vi "3_ReadDatatoWaveform.vi"(8 "error in (no error)":errorcluster, 11 "file path (IN)":path) -> (0 "error out":errorcluster, 2 "Waveform Graph":waveform(dbl)[](graph), 3 "file path (OUT)":path, 4 "dt":dbl, 5 "Ch 2 Data":dbl[](array[numeric]), 6 "Ch 3 Data":dbl[](array[numeric]), 7 "Ch 1 Data":dbl[](array[numeric]))   [LabVIEW 2020]
uses:
  <vilib>/Utility/file.llb/Read Delimited Spreadsheet (string).vi
  <vilib>/Utility/file.llb/Read Delimited Spreadsheet (DBL).vi
panel:
  out "Spread Sheet Display":string[][](array[string])
  out "Data Display":dbl[][](array[numeric])
  # "Channel 1"
  # "Channel 2"
  # "Channel 3"
  # "C:\\Users\\zbmbdt\\Desktop\\Assignment\\Project1_AC Module\\LabVIEW_Project_AC_Module\\1_ALL_VI\\GRAPH_11_30\\graphdata.csv"
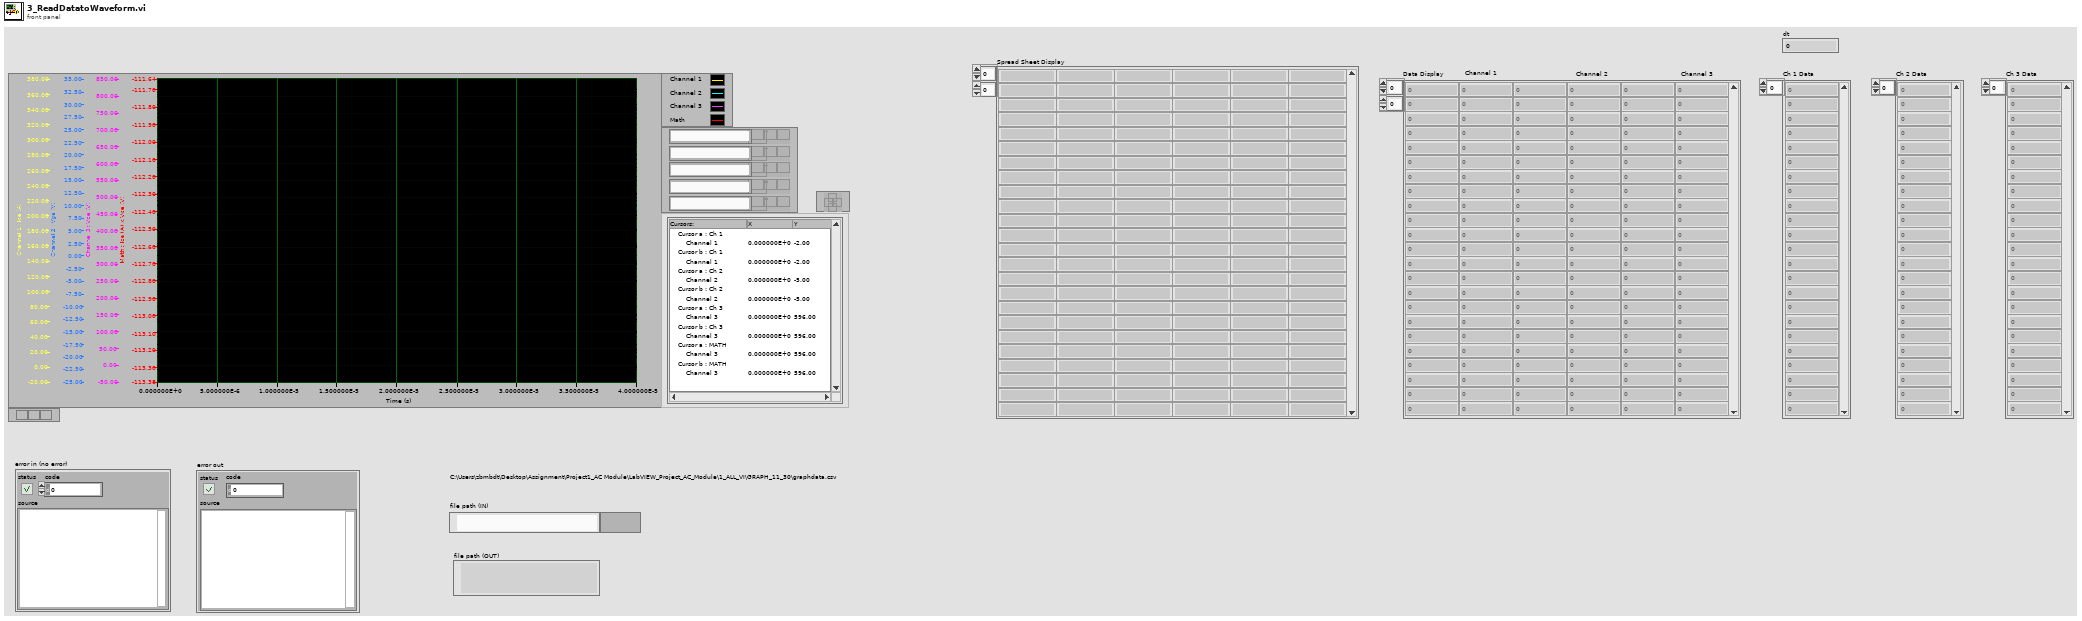
[diagram p1: front panel]
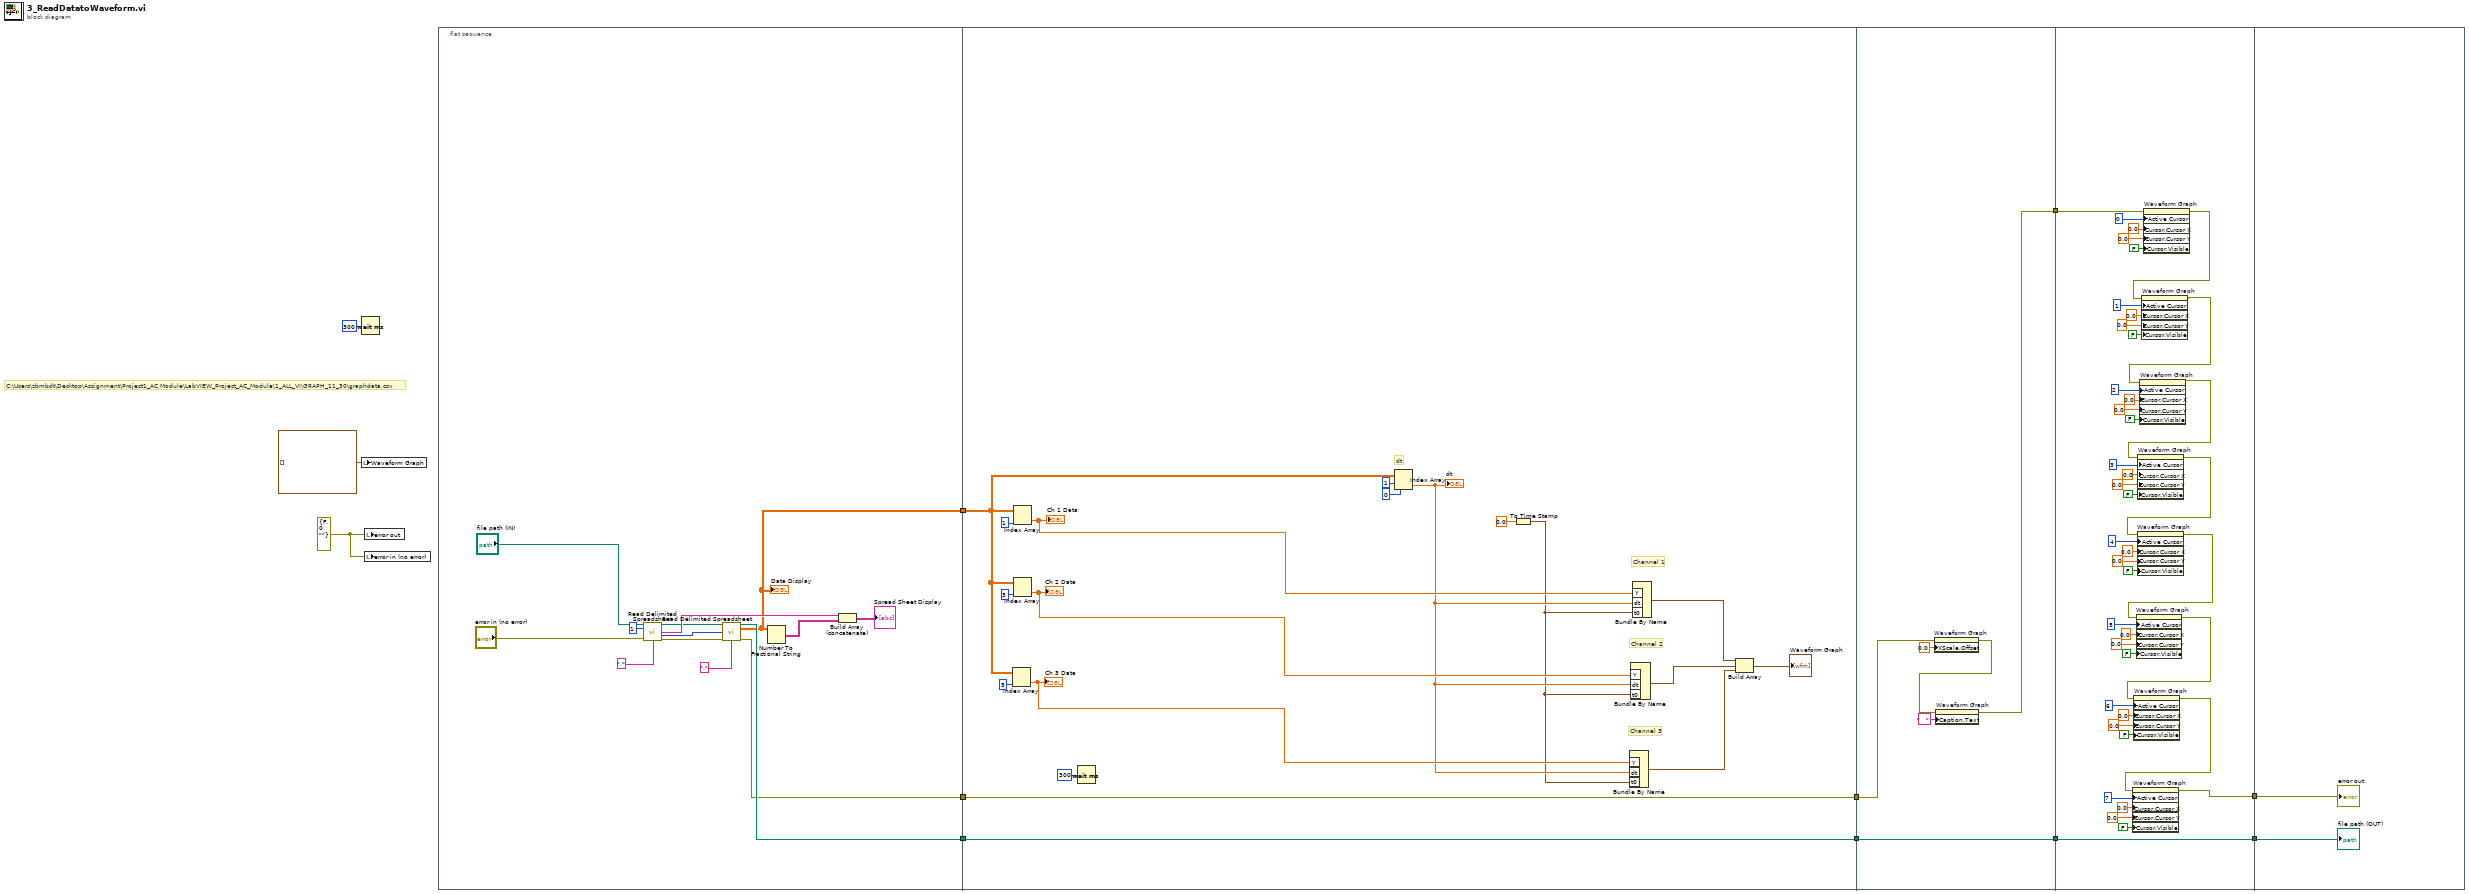
[diagram p0: block diagram]
diagram:
  w2 = errorcluster {"status"=FALSE, "code"=0, "source"=""} ("error out")
  # "C:\\Users\\zbmbdt\\Desktop\\Assignment\\Project1_AC Module\\LabVIEW_Project_AC_Module\\1_ALL_VI\\GRAPH_11_30\\graphdata.csv"
  n1 = Wait (ms)(milliseconds to wait=u32 300) -> ()  [unwired: 1 out]
  n2 = local write "Waveform Graph"(waveform(dbl)[] [] ("Waveform Graph")) -> ()
  n3 = local write "error out"(w2) -> ()
  n4 = local write "error in (no error)"(w2) -> ()
  n5 = flat-sequence {
    tunnel: [w14] -> w7
    tunnel: [w13] -> w6
    tunnel: [w15] -> w5
    tunnel: [w31] -> w12
    tunnel: [w30] -> w11
    tunnel: w7 -> [w36]
    tunnel: w6 -> [w31]
    tunnel: w5 -> [w30]
    tunnel: w12 -> [w50]
    tunnel: w11 -> [w51]
    tunnel: [w51] -> w10
    tunnel: [w47] -> w9
    tunnel: w10 -> [w93]
    tunnel: [w93] -> w4
    tunnel: w9 -> [w92]
    tunnel: [w52] -> w3
    tunnel: w4 -> [w95]
    tunnel: w3 -> [w94]
    frame #0 {
      n6 = call-poly <vilib>:"Read Delimited Spreadsheet.vi"("file path (dialog if empty)"="file path (IN)", "number of rows (all:-1)"=1, "error in (no error)"="error in (no error)", "delimiter (\\t)"="," ("delimiter (\\t)")) -> ("new file path (Not A Path if cancelled)"=w20:path, "first row"=w21:string[], "mark after read (chars.)"=w19:i32, "error out"=w25:errorcluster)  [unwired: 6 in, 2 out]
      n7 = call-poly <vilib>:"Read Delimited Spreadsheet.vi"("file path (dialog if empty)"=w20, "start of read offset (chars.:0)"=w19, "error in (no error)"=w25, "delimiter (\\t)"="," ("delimiter (\\t)")) -> ("new file path (Not A Path if cancelled)"=w15:path, "all rows"=w14:dbl[][], "error out"=w13:errorcluster)  [unwired: 6 in, 3 out]
      "Data Display" <- w14
      n8 = Number To Fractional String(number=w14) -> (F-format string=w22:string[][])  [unwired: 3 in]
      n9 = Build Array (concatenate)(w21, w22) -> (→"Spread Sheet Display":string[][])
    }
    frame #1 {
      # "dt"
      # "Channel 3"
      # "Channel 2"
      # "Channel 1"
      n10 = Index Array(array=w36, index (col)=5 ("disabled index (col)")) -> (element=w37:dbl[])  [unwired: 1 in]
      "Ch 3 Data" <- w37
      n11 = Index Array(array=w36, index (col)=1 ("disabled index (col)")) -> (element=w39:dbl[])  [unwired: 1 in]
      "Ch 1 Data" <- w39
      n12 = Index Array(array=w36, index (col)=3 ("disabled index (col)")) -> (element=w38:dbl[])  [unwired: 1 in]
      "Ch 2 Data" <- w38
      n13 = Wait (ms)(milliseconds to wait=u32 300) -> ()  [unwired: 1 out]
      n14 = Index Array(array=w36, index (row)=1, index (col)=0 ("disabled index (col)")) -> (element=w33:dbl)
      "dt" <- w33
      n15 = To Time Stamp(1:0.0 ("number")) -> (0:w28:timestamp)
      n16 = Bundle By Name("Y"=w37, "dt"=w33, "t0"=w28) -> (w40:waveform(dbl))  [unwired: 1 in]
      n17 = Bundle By Name("Y"=w38, "dt"=w33, "t0"=w28) -> (w41:waveform(dbl))  [unwired: 1 in]
      n18 = Bundle By Name("Y"=w39, "dt"=w33, "t0"=w28) -> (w42:waveform(dbl))  [unwired: 1 in]
      n19 = Build Array(w42, w41, w40) -> (→"Waveform Graph":waveform(dbl)[])
    }
    frame #2 {
      n20 = property on="Waveform Graph" class="WFGraph (strict)"(error in=w50, "XScale.Offset"=0.0 ("X Scale.Offset and Multiplier:Offset")) -> (error out=w48:errorcluster)  [unwired: 1 in, 1 out]
      n21 = property on="Waveform Graph" class="WFGraph (strict)"(error in=w48, "Caption.Text"="   ") -> (error out=w47:errorcluster)  [unwired: 1 in, 1 out]
    }
    frame #3 {
      n22 = property on="Waveform Graph" class="WFGraph (strict)"(error in=w92, "Active Cursor"=u32 0, "Cursor.Cursor X"=0.0 ("Cursor.Cursor Position:Cursor X"), "Cursor.Cursor Y"=0.0 ("Cursor.Cursor Position:Cursor Y"), "Cursor.Visible"=FALSE) -> (error out=w59:errorcluster)  [unwired: 1 in, 1 out]
      n23 = property on="Waveform Graph" class="WFGraph (strict)"(error in=w59, "Active Cursor"=u32 1, "Cursor.Cursor X"=0.0 ("Cursor.Cursor Position:Cursor X"), "Cursor.Cursor Y"=0.0 ("Cursor.Cursor Position:Cursor Y"), "Cursor.Visible"=FALSE) -> (error out=w58:errorcluster)  [unwired: 1 in, 1 out]
      n24 = property on="Waveform Graph" class="WFGraph (strict)"(error in=w58, "Active Cursor"=u32 2, "Cursor.Cursor X"=0.0 ("Cursor.Cursor Position:Cursor X"), "Cursor.Cursor Y"=0.0 ("Cursor.Cursor Position:Cursor Y"), "Cursor.Visible"=FALSE) -> (error out=w57:errorcluster)  [unwired: 1 in, 1 out]
      n25 = property on="Waveform Graph" class="WFGraph (strict)"(error in=w57, "Active Cursor"=u32 3, "Cursor.Cursor X"=0.0 ("Cursor.Cursor Position:Cursor X"), "Cursor.Cursor Y"=0.0 ("Cursor.Cursor Position:Cursor Y"), "Cursor.Visible"=FALSE) -> (error out=w56:errorcluster)  [unwired: 1 in, 1 out]
      n26 = property on="Waveform Graph" class="WFGraph (strict)"(error in=w56, "Active Cursor"=u32 4, "Cursor.Cursor X"=0.0 ("Cursor.Cursor Position:Cursor X"), "Cursor.Cursor Y"=0.0 ("Cursor.Cursor Position:Cursor Y"), "Cursor.Visible"=FALSE) -> (error out=w55:errorcluster)  [unwired: 1 in, 1 out]
      n27 = property on="Waveform Graph" class="WFGraph (strict)"(error in=w55, "Active Cursor"=u32 5, "Cursor.Cursor X"=0.0 ("Cursor.Cursor Position:Cursor X"), "Cursor.Cursor Y"=0.0 ("Cursor.Cursor Position:Cursor Y"), "Cursor.Visible"=FALSE) -> (error out=w54:errorcluster)  [unwired: 1 in, 1 out]
      n28 = property on="Waveform Graph" class="WFGraph (strict)"(error in=w54, "Active Cursor"=u32 6, "Cursor.Cursor X"=0.0 ("Cursor.Cursor Position:Cursor X"), "Cursor.Cursor Y"=0.0 ("Cursor.Cursor Position:Cursor Y"), "Cursor.Visible"=FALSE) -> (error out=w53:errorcluster)  [unwired: 1 in, 1 out]
      n29 = property on="Waveform Graph" class="WFGraph (strict)"(error in=w53, "Active Cursor"=u32 7, "Cursor.Cursor X"=0.0 ("Cursor.Cursor Position:Cursor X"), "Cursor.Cursor Y"=0.0 ("Cursor.Cursor Position:Cursor Y"), "Cursor.Visible"=FALSE) -> (error out=w52:errorcluster)  [unwired: 1 in, 1 out]
    }
    frame #4 {
      "error out" <- w94
      "file path (OUT)" <- w95
    }
  }
